vi "IntakeDashReadNetwork.vi"() -> (0 "HaveCoralSensor":bool, 1 "MotorDmdRight":dbl, 2 "MotorDmdLeft":dbl, 3 "MotorDmdTop":dbl, 4 "HaveAlgaeSensor":bool, 6 "CurrentState":T1)   [LabVIEW 2023]
doc: "Writes motor demand and sensor data to the Dashboard."
uses:
  IntakeStates.ctl
  <vilib>/Rock Robotics/Network Tables/NT Read Boolean.vi
  <vilib>/Rock Robotics/Network Tables/NT Read Number.vi
  IntakeGlobal.vi
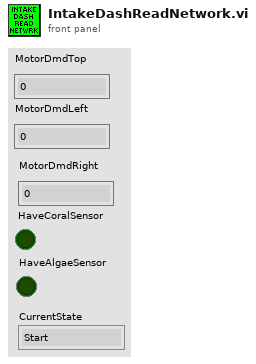
[diagram p1: front panel]
types:
  T1 = typedef "IntakeStates.ctl" = enum16{"Start", "WaitForCommand", "IntakeCoral", "IntakeAlgae", "WaitForCoral", "WaitForAlgae", "DepositCoral", "DepositAlgae", "DepositCoralTimer", "DepositAlgaeTimer"}
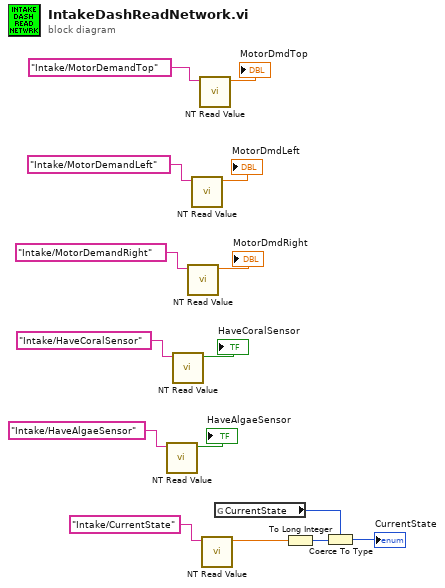
[diagram p0: block diagram]
diagram:
  n1 = call-poly <vilib>:"NT Read Value.vi"("name"="Intake/HaveAlgaeSensor") -> ("value"=→"HaveAlgaeSensor":bool)  [unwired: 8 in, 2 out]
  n2 = call-poly <vilib>:"NT Read Value.vi"("name"="Intake/HaveCoralSensor") -> ("value"=→"HaveCoralSensor":bool)  [unwired: 8 in, 2 out]
  n3 = call-poly <vilib>:"NT Read Value.vi"("name"="Intake/MotorDemandRight") -> ("value"=→"MotorDmdRight":dbl)  [unwired: 8 in, 2 out]
  n4 = call-poly <vilib>:"NT Read Value.vi"("name"="Intake/MotorDemandLeft") -> ("value"=→"MotorDmdLeft":dbl)  [unwired: 8 in, 2 out]
  n5 = call-poly <vilib>:"NT Read Value.vi"("name"="Intake/MotorDemandTop") -> ("value"=→"MotorDmdTop":dbl)  [unwired: 8 in, 2 out]
  n6 = call-poly <vilib>:"NT Read Value.vi"("name"="Intake/CurrentState") -> ("value"=w4:dbl)  [unwired: 8 in, 2 out]
  n7 = global read "IntakeGlobal.vi" "CurrentState"() -> (w2:T1)
  n8 = To Long Integer(number=w4) -> (32bit integer=w3:i32)
  n9 = Coerce To Type(0:w3, 1:w2) -> (2:→"CurrentState":T1)
